vi "test load graph and plot t90.vi"() -> ()   [LabVIEW 2019]
uses:
  Controls/JSON - GetData.ctl
  Controls/JSON - Report.ctl
  <vilib>/httpClient/POSTBuffer.vi
  <userlib>/_OpenG.lib/array/array.llb/Remove Duplicates from 1D Array (String)__ogtk.vi
  <userlib>/_OpenG.lib/array/array.llb/Delete Elements from 1D Array (String)__ogtk.vi
  <vilib>/httpClient/LabVIEWHTTPClient.lvlib
  <vilib>/Analysis/NI_AALPro.lvlib
panel:
  out "testname":string[](array[string])
  out "testtype":string[](array[string])
  out "Image":T1(plugin-control)
  out "empty picture":picture
  out "standard error":string
  out "standard output":string
  out "concatenated string":string
  out "Height Settlement":string
  out "Sqrt Minute":string
  out "XY 2":cluster{"Array out":dbl[], "Array out":dbl[]}[](graph)
  out "Height Settlement":dbl[](array[numeric])
  out "Minute":dbl[](array[numeric])
  out "Sqrt Minute":dbl[](array[numeric])
  out "number":dbl[][](array[numeric])
  out "XY":cluster{"Array out":dbl[], "Array out":dbl[]}[](graph)
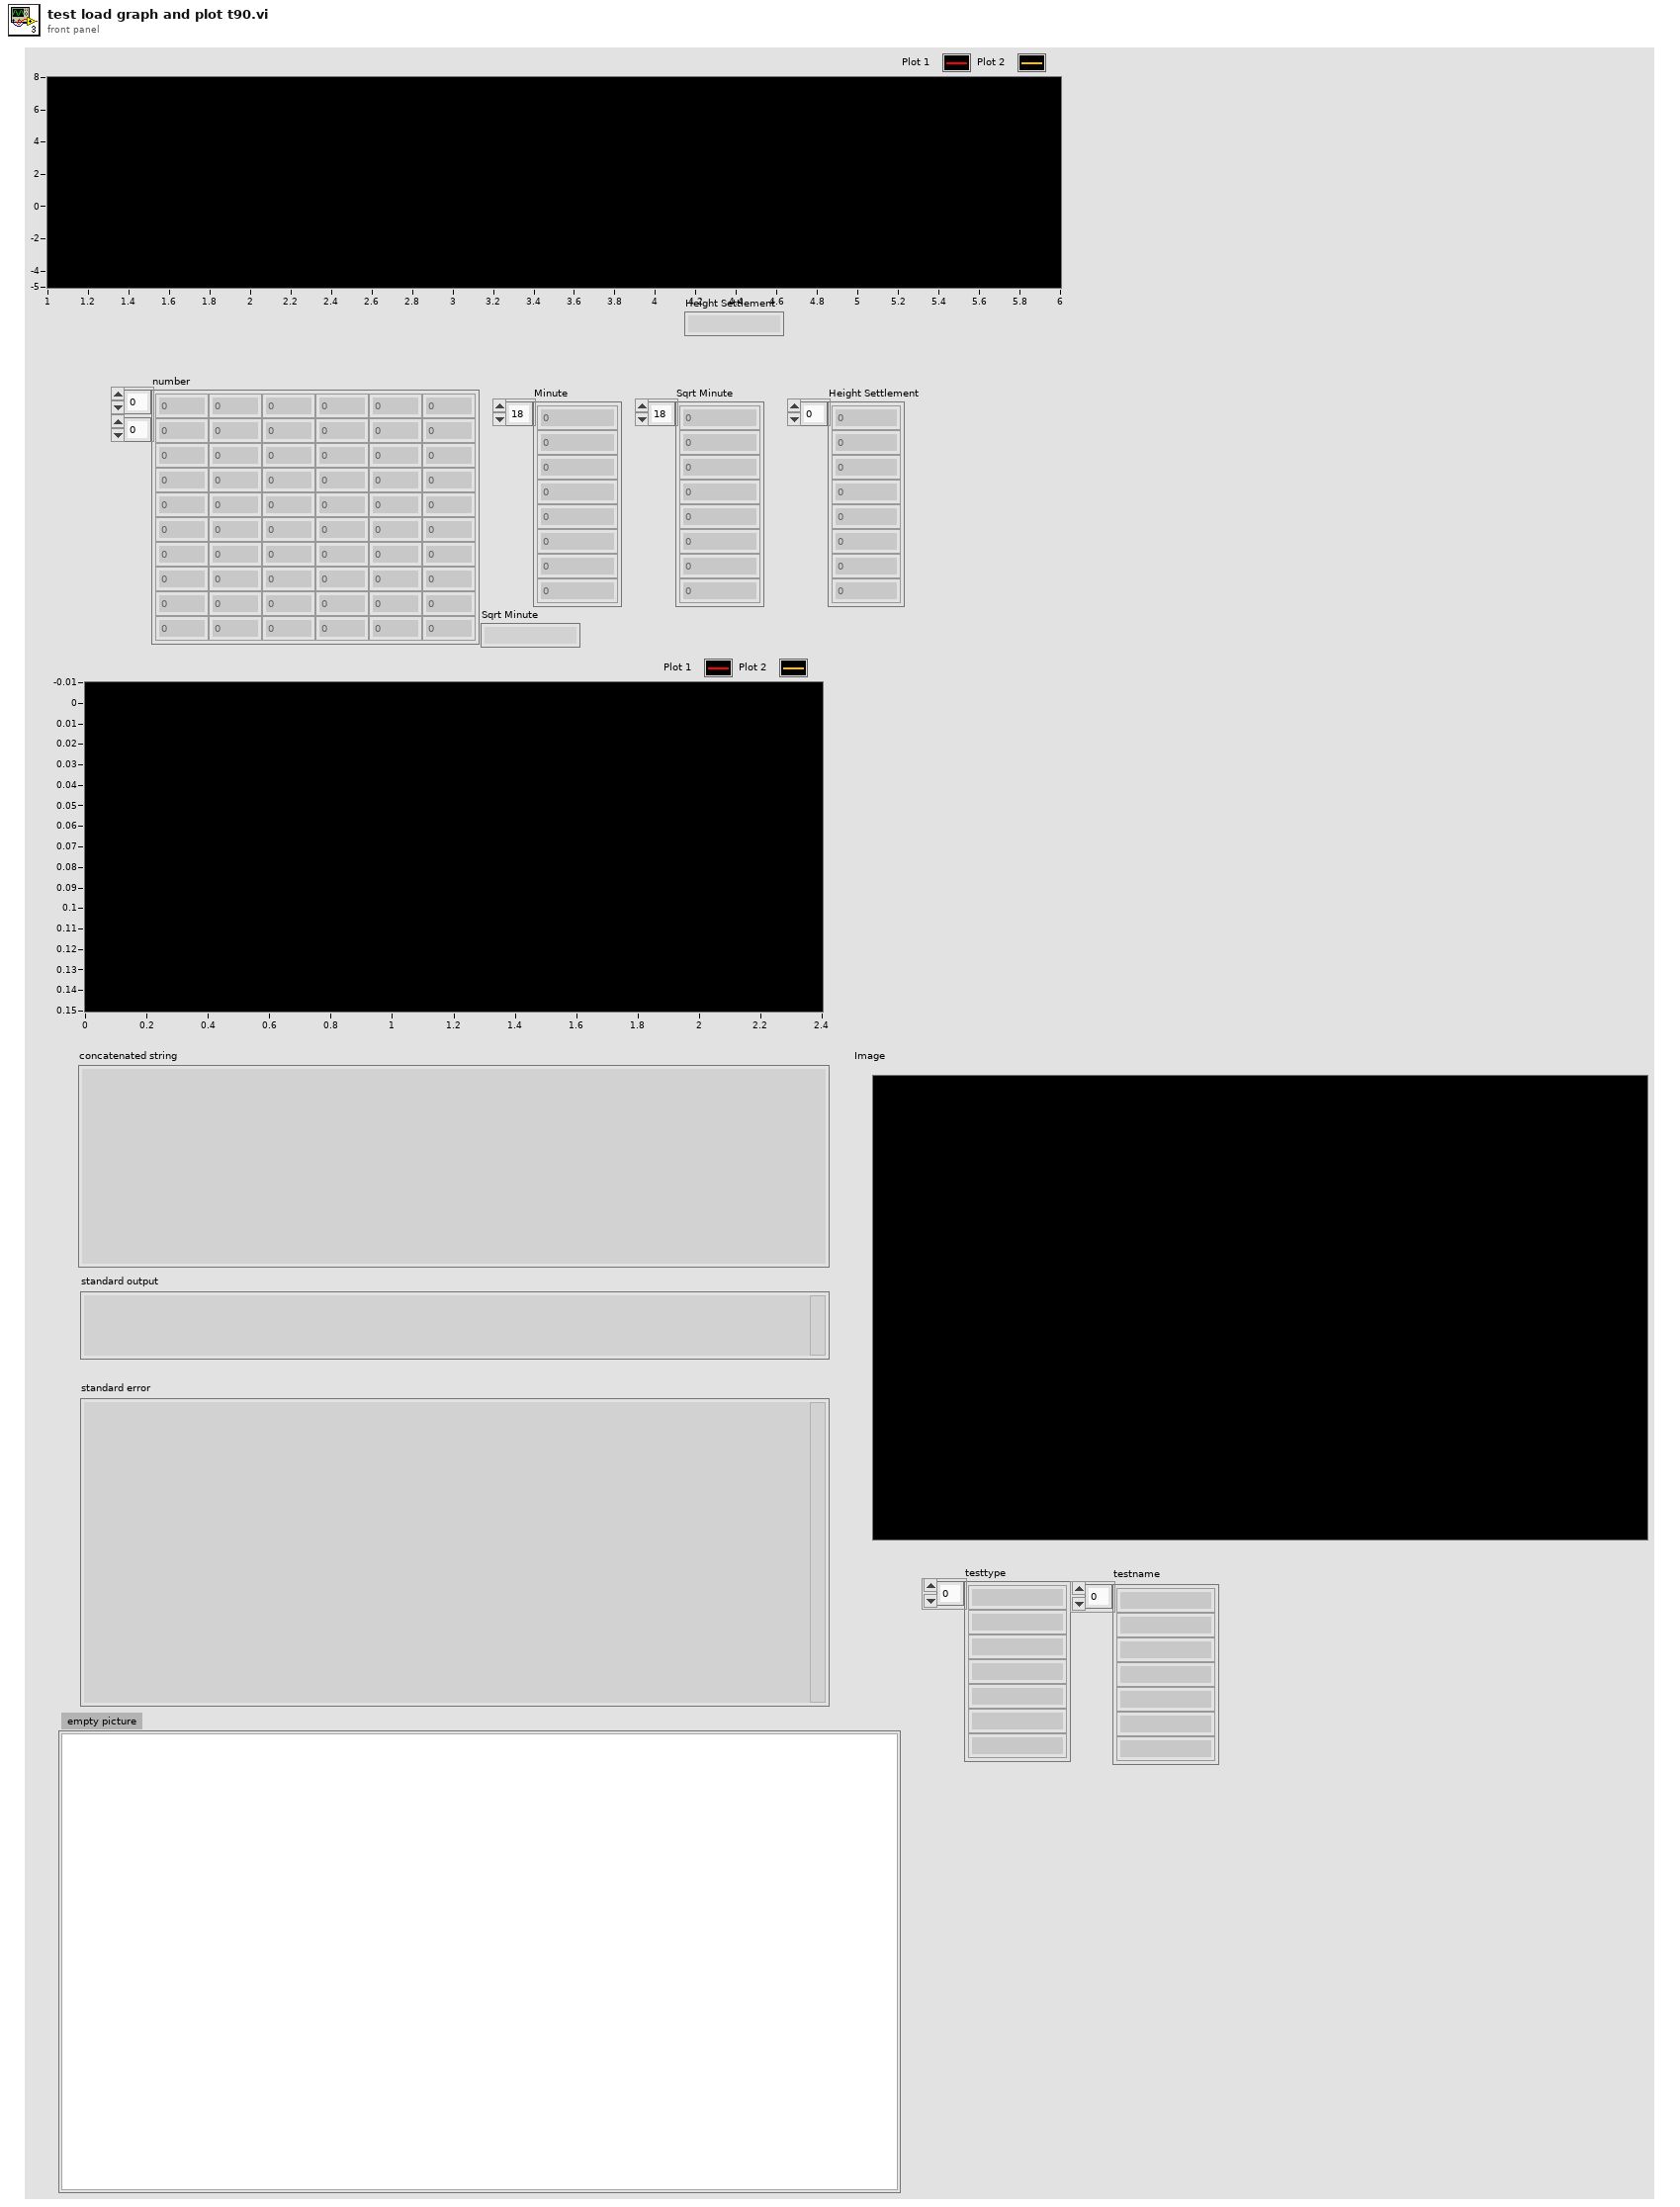
[diagram p1: front panel]
types:
  T1 = typedef "IMAQ Image.ctl" = refnum<image>
  T2 = typedef "Image Type" = u32
  T3 = typedef "JSON - GetData.ctl" = cluster{"status":string, "data":cluster{"timestamp":string, "elapsetime":string, "testname":string, "testtype":u16, "data":string[]}[]}
  T4 = cluster{"testtype":u16, "testname":string, "fileid":string}
  T5 = typedef "JSON - Report.ctl" = cluster{"status":string, "data":cluster{"testname":string, "testtype":string}[]}
  T6 = cluster{"timestamp":string, "elapsetime":string, "testname":string, "testtype":u16, "data":string[]}[]
  T7 = typedef "imagedata.ctl" = cluster{"image type":i32, "image depth":i32, "image":u8[], "mask":u8[], "colors":u32[], "Rectangle":cluster{"left":i16, "top":i16, "right":i16, "bottom":i16}}
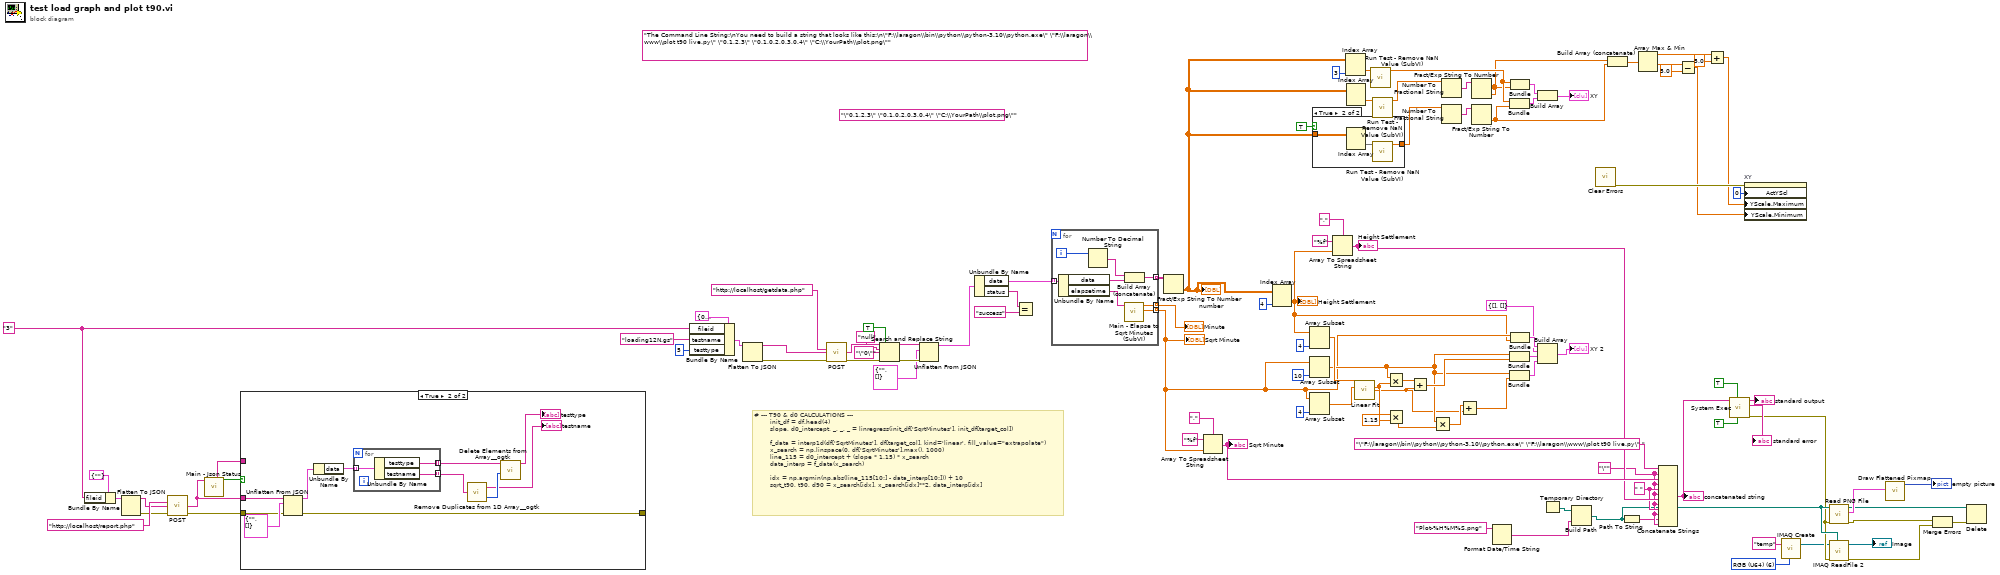
[diagram p0: block diagram]
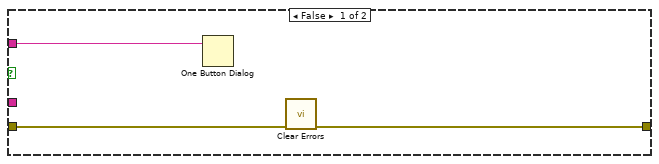
[diagram p2: hidden frame]
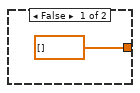
[diagram p3: hidden frame]
diagram:
  w16 = T2 6 items=["Grayscale (U8)", "Grayscale (I16)", "Grayscale (SGL)", "Complex (CSG)", "RGB (U32)", "HSL (U32)", "RGB (U64)", "Grayscale (U16)"] ("Image Type")
  w33 = " " ("string")
  w32 = "\"" ("string")
  (unwired) "\"0,1,2,3\" \"0.1,0.2,0.3,0.4\" \"C:\\YourPath\\plot.png\"" ("y")
  (unwired) "The Command Line String:\nYou need to build a string that looks like this:\n\"F:\\laragon\\bin\\python\\python-3.10\\python.exe\" \"F:\\laragon\\www\\plot t90 live.py\" \"0,1,2,3\" \"0.1,0.2,0.3,0.4\" \"C:\\YourPath\\plot.png\"" ("y")
  w1 = "3" ("fileid")
  # "# --- T90 & d0 CALCULATIONS ---\n        init_df = df.head(4)\n        slope, d0_intercept, _, _, _ = linregress(init_df['SqrtMinutes'], init_df[target_col])\n        \n        f_data = interp1d(df['SqrtMinutes'], df[target_col], kind='linear', fill_value=\"extrapolate\")\n        x_search = np.linspace(0, df['SqrtMinutes'].max(), 1000)\n        line_115 = d0_intercept + (slope * 1.15) * x_search\n        data_interp = f_data(x_search)\n        \n        idx = np.argmin(np.abs(line_115[10:] - data_interp[10:])) + 10\n        sqrt_t90, t90, d90 = x_search[idx], x_search[idx]**2, data_interp[idx]"
  n1 = Bundle By Name(cluster=cluster{"fileid":string} {"fileid"=""}, "fileid"=w1) -> (w9:cluster{"fileid":string})
  n2 = Flatten To JSON(anything=w9) -> (JSON string=w6:string, 11:w7:errorcluster)  [unwired: 2 in]
  n3 = call-poly <vilib>:"POST.vi"("url"="http://localhost/report.php", "buffer"=w6, "error in (no error)"=w7) -> ("body"=w4:string, "error out"=w5:errorcluster)  [unwired: 9 in, 2 out]
  n4 = call "Main - Json Status.vi"("json"=w4) -> ("Success?"=w3:bool, "message"=w2:string)  [unwired: 9 in]
  n5 = case shown="True" w3 {
    tunnel: w5 -> [w109 w120]
    tunnel: [w108 w112] -> _
    tunnel: w4 -> [_ w111]
    tunnel: w2 -> [w110 _]
    frame False {
      n6 = One Button Dialog(message=w110) -> ()  [unwired: 1 in, 1 out]
      n7 = call <vilib>:"Clear Errors.vi"("error in (no error)"=w109) -> ("error out"=w108:errorcluster)  [unwired: 5 in, 1 out]
    }
    frame True {
      n8 = Unflatten From JSON(JSON string=w111, type and defaults=T5 {"status"="", "data"=[]}, error in (no error)=w120) -> (value=w118:T5, error out=w112:errorcluster)  [unwired: 4 in]
      n9 = Unbundle By Name(w118) -> ("data"=w119:cluster{"testname":string, "testtype":string}[])
      n10 = for {
        tunnel: w119 -> [w124] mode=indexing
        tunnel: [w123] -> w115 mode=indexing
        tunnel: [w122] -> w116 mode=indexing
        n11 = Unbundle By Name(w124) -> ("testtype"=w123:string, "testname"=w122:string)
      }
      n12 = call-poly <userlib>:"Remove Duplicates from 1D Array__ogtk.vi"("Input Array"=w116) -> ("Output Array"=→"testname":string[], "indices of removed elements"=w117:i32[])
      n13 = call-poly <userlib>:"Delete Elements from Array__ogtk.vi"("indices"=w117, "array"=w115) -> ("array w/ subset deleted"=→"testtype":string[])  [unwired: 8 in, 1 out]
    }
  }
  n14 = Bundle By Name(cluster=T4 {"testtype"=0, "testname"="", "fileid"=""}, "fileid"=w1, "testname"="loading12N.gs", "testtype"=u16 5) -> (w107:T4)
  n15 = Flatten To JSON(anything=w107) -> (JSON string=w106:string, 11:w93:errorcluster)  [unwired: 2 in]
  n16 = call-poly <vilib>:"POST.vi"("url"="http://localhost/getdata.php", "buffer"=w106, "error in (no error)"=w93) -> ("body"=w102:string, "error out"=w92:errorcluster)  [unwired: 9 in, 2 out]
  n17 = Search and Replace String(replace all?=TRUE ("replace all? (F)"), input string=w102, search string="null", replace string="\"0\"" ("replace string (\"\")"), error in=w92) -> (result string=w101:string, error out=w103:errorcluster)  [unwired: 3 in, 2 out]
  n18 = Unflatten From JSON(JSON string=w101, type and defaults=T3 {"status"="", "data"=[]}, error in (no error)=w103) -> (value=w104:T3)  [unwired: 4 in, 1 out]
  n19 = Unbundle By Name(w104) -> ("data"=w70:T6, "status"=w105:string)
  n20 = Equal?(x=w105, y="success") -> ()  [unwired: 1 out]
  n21 = for {
    tunnel: w70 -> [w132] mode=indexing
    tunnel: [w130] -> w91 mode=indexing
    tunnel: [w126] -> w64 mode=indexing
    tunnel: [w125] -> w42 mode=indexing
    i -> [w128]
    n22 = Unbundle By Name(w132) -> ("data"=w131:string[], "elapsetime"=w127:string)
    n23 = Number To Decimal String(number=w128) -> (decimal integer string=w129:string)  [unwired: 1 in]
    n24 = call "Main - Elapse to Sqrt Minutes (SubVI).vi"("Elapse"=w127) -> ("sqrt (Minute)"=w125:dbl, "Minute"=w126:dbl)  [unwired: 9 in]
    n25 = Build Array (concatenate)(w129, w131) -> (w130:string[])
  }
  "Sqrt Minute" <- w42
  "Minute" <- w64
  n26 = Fract/Exp String To Number(string=w91) -> (number=w63:dbl[][])  [unwired: 3 in, 1 out]
  "number" <- w63
  n27 = Array To Spreadsheet String(delimiter (Tab)=",", array=w42, 3:"%f" ("format string")) -> (spreadsheet string=w35:string)
  "Sqrt Minute" <- w35
  n28 = Index Array(array=w63, index (col)=4 ("disabled index (col)")) -> (element=w37:dbl[])  [unwired: 1 in]
  "Height Settlement" <- w37
  n29 = Array Subset(array=w37, length=4) -> (w57:dbl[])  [unwired: 1 in]
  n30 = Array Subset(array=w42, length=10) -> (w46:dbl[])  [unwired: 1 in]
  n31 = Array Subset(array=w42, length=4) -> (w56:dbl[])  [unwired: 1 in]
  n32 = case shown="True" TRUE {
    tunnel: [dbl[] [] w136] -> w83
    tunnel: w63 -> [_ w135]
    frame False {
    }
    frame True {
      n33 = Index Array(array=w135) -> (element=w134:dbl[])  [unwired: 2 in]
      n34 = call "Run Test - Remove NaN Value (SubVI).vi"("Array"=w134) -> ("Array out"=w136:dbl[])  [unwired: 10 in]
    }
  }
  n35 = Array To Spreadsheet String(delimiter (Tab)=",", array=w37, 3:"%f" ("format string")) -> (spreadsheet string=w34:string)
  "Height Settlement" <- w34
  n36 = Index Array(array=w63, index (col)=3 ("disabled index (col)")) -> (element=w69:dbl[])  [unwired: 1 in]
  n37 = Index Array(array=w63) -> (element=w68:dbl[])  [unwired: 2 in]
  n38 = call <vilib>:"Linear Fit.vi"("Y"=w57, "X"=w56) -> ("slope"=w51:dbl, "intercept"=w44:dbl)  [unwired: 9 in, 3 out]
  n39 = call "Run Test - Remove NaN Value (SubVI).vi"("Array"=w69) -> ("Array out"=w87:dbl[])  [unwired: 10 in]
  n40 = call "Run Test - Remove NaN Value (SubVI).vi"("Array"=w68) -> ("Array out"=w85:dbl[])  [unwired: 10 in]
  n41 = Multiply(x=w46, y=w51) -> (x*y=w54:dbl[])
  n42 = Multiply(x=w51, y=1.15) -> (x*y=w49:dbl)
  n43 = Add(x=w54, y=w44) -> (x+y=w52:dbl[])
  n44 = Multiply(x=w46, y=w49) -> (x*y=w45:dbl[])
  n45 = Number To Fractional String(number=w85) -> (F-format string=w86:string[])  [unwired: 3 in]
  n46 = Number To Fractional String(number=w83) -> (F-format string=w84:string[])  [unwired: 3 in]
  n47 = Add(x=w45, y=w44) -> (x+y=w43:dbl[])
  n48 = Fract/Exp String To Number(string=w86) -> (number=w73:dbl[])  [unwired: 3 in, 1 out]
  n49 = Fract/Exp String To Number(string=w84) -> (number=w74:dbl[])  [unwired: 3 in, 1 out]
  n50 = Format Date/Time String(time format string (%c)="Plot-%H%M%S.png") -> (date/time string=w29:string)  [unwired: 2 in]
  n51 = Bundle("Array out"=w87, w74) -> (w89:cluster{"Array out":dbl[], dbl[]})  [unwired: 1 in]
  n52 = Bundle(w46, w52) -> (w48:cluster{dbl[], dbl[]})  [unwired: 1 in]
  n53 = Bundle(w46, w43) -> (w47:cluster{dbl[], dbl[]})  [unwired: 1 in]
  n54 = Bundle("Array out"=w87, w73) -> (w90:cluster{"Array out":dbl[], dbl[]})  [unwired: 1 in]
  n55 = Bundle(w42, w37) -> (w58:cluster{dbl[], dbl[]})  [unwired: 1 in]
  n56 = Build Array(w90, w89) -> (→"XY":cluster{"Array out":dbl[], dbl[]}[])
  n57 = Build Array(w58, cluster{dbl[], "Best Linear Fit":dbl[]} {[], "Best Linear Fit"=[]} ("element"), w48, w47) -> (→"XY 2":cluster{dbl[], "Best Linear Fit":dbl[]}[])
  n58 = Temporary Directory() -> (w31:path)
  n59 = Build Path(base path=w31, name or relative path=w29) -> (appended path=w19:path)
  n60 = call <vilib>:"Clear Errors.vi"() -> ("error out"=w82:errorcluster)  [unwired: 6 in, 1 out]
  n61 = Build Array (concatenate)(w73, w74) -> (w72:dbl[])
  n62 = Path To String(path=w19) -> (string=w28:string)
  n63 = Array Max & Min(array=w72) -> (max value=w80:dbl, min value=w77:dbl)  [unwired: 2 out]
  n64 = Concatenate Strings("\"F:\\laragon\\bin\\python\\python-3.10\\python.exe\" \"F:\\laragon\\www\\plot t90 live.py\" " ("y"), w32, w35, w32, w33, w32, w34, w32, w33, w32, w28, w32) -> (w23:string)
  "concatenated string" <- w23
  n65 = Subtract(x=w77, y=5.0) -> (x-y=w76:dbl)
  n66 = Add(x=w80, y=5.0) -> (x+y=w79:dbl)
  n67 = call <vilib>:"System Exec.vi"("run minimized? (F)"=TRUE, "wait until completion? (T)"=TRUE, "command line"=w23) -> ("error out"=w18:errorcluster, "standard error"=→"standard error":string, "standard output"=→"standard output":string)  [unwired: 5 in, 1 out]
  n68 = property on="XY" class="XYGraph (strict)"(error in=w82, "ActYScl"=0 ("Active Y Scale"), "YScale.Maximum"=w79, "YScale.Minimum"=w76) -> ()  [unwired: 1 in, 2 out]
  n69 = call "IMAQ Create"("Image Name"="temp", "Image Type"=w16) -> ("New Image"=w17:T1)  [unwired: 3 in, 1 out]
  n70 = call <vilib>:"Read PNG File.vi"("error in (no error)"=w18, "path to PNG file"=w19) -> ("error out"=w14:errorcluster, "image data"=w22:T7, "path"=w20:path)  [unwired: 7 in]
  n71 = call "IMAQ ReadFile 2"("File Path"=w19, "error in (no error)"=w18, "Image"=w17) -> ("error out"=w13:errorcluster, "Image Out"=→"Image":T1)  [unwired: 4 in, 3 out]
  n72 = call <vilib>:"Draw Flattened Pixmap.vi"("image data"=w22) -> ("new picture"=→"empty picture":picture)  [unwired: 8 in]
  n73 = Merge Errors(w14, w13) -> (w12:errorcluster)
  n74 = Delete(path (use dialog)=w20, error in=w12) -> ()  [unwired: 3 in, 3 out]
